vi "Get guard interval.vi"(8 "error in (no error)":errorcluster, 11 "niDTS WLAN Dut Data in":refnum<class "niDTS WLAN Dut Data.lvclass">) -> (0 "error out":errorcluster, 2 "guard interval":cluster{"Value":T1, "Init":bool}, 3 "niDTS WLAN Dut Data out":refnum<class "niDTS WLAN Dut Data.lvclass">)   [LabVIEW 2015, in "niDTS WLAN.lvlib" / "niDTS WLAN Dut Data.lvclass"]
uses:
  niDTS WLAN Dut Data.lvclass
  Includes/niDTS WLAN INC GI.ctl
  niDTS WLAN Dut Data.lvclass/niDTS WLAN Dut Data.ctl
  niDTS WLAN.lvlib
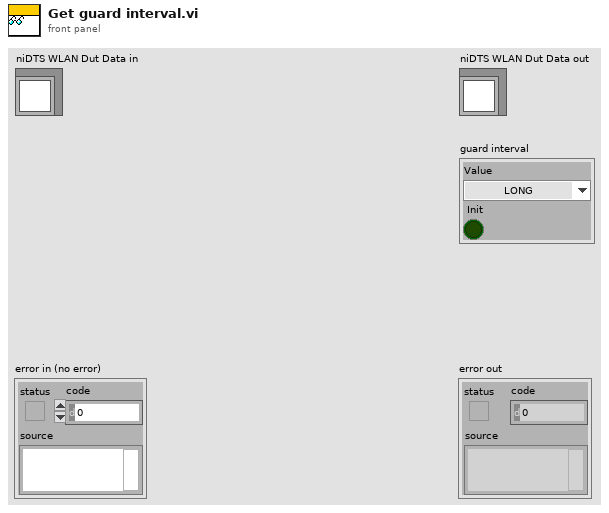
[diagram p1: front panel]
types:
  T1 = typedef "niDTS WLAN.lvlib/niDTS WLAN INC GI.ctl" = enum16{"LONG", "SHORT"}
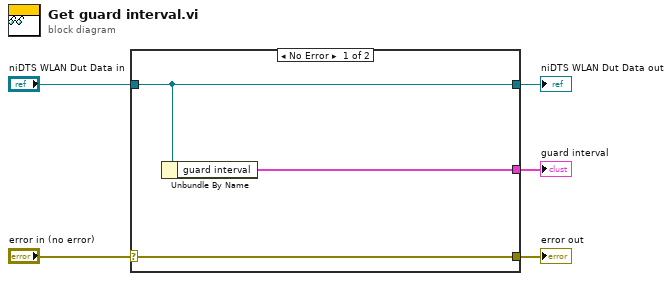
[diagram p0: block diagram]
diagram:
  n1 = case shown="No Error" "error in (no error)" {
    selector: "error in (no error)" -> [w8 w9]
    tunnel: [w8 w9] -> w4
    tunnel: [w7 w10] -> w2
    tunnel: "niDTS WLAN Dut Data in" -> [w7 w10]
    tunnel: [w6 _] -> w1
    frame No Error {
      n2 = Unbundle By Name(w7) -> ("guard interval"=w6:cluster{"Value":T1, "Init":bool})
    }
    frame Error {
    }
  }
  "error out" <- w4
  "niDTS WLAN Dut Data out" <- w2
  "guard interval" <- w1
